vi "Get App Paths.vi"(8 "error in (no error)":errorcluster, 11 "Build Name":string) -> (0 "error out":errorcluster, 3 "Paths":T1)   [LabVIEW 2020, in "RTAF.lvlib"]
doc: "This VI returns the root directory of the main VI.\n\nIf the system is running as an executable it returns the directory the exe resides in."
uses:
  RTAF.lvlib
  App Paths.ctl
  <userlib>/_OpenG.lib/file/file.llb/Convert File Extension (Path)__ogtk.vi
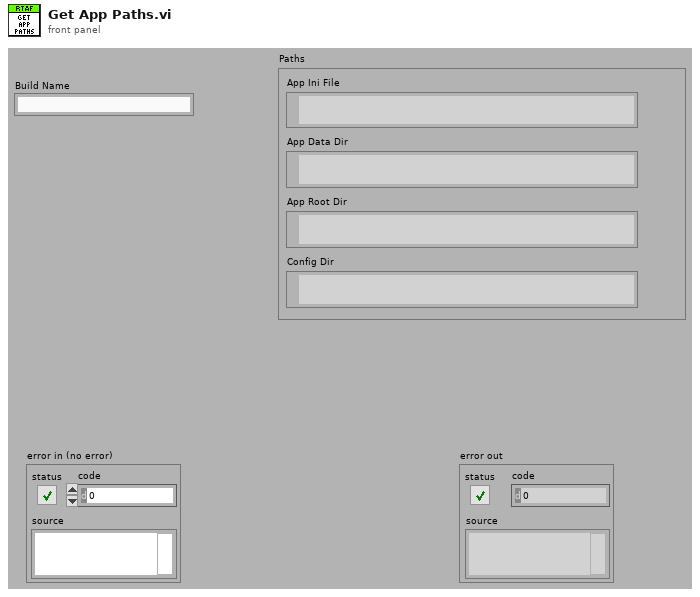
[diagram p1: front panel]
types:
  T1 = typedef "RTAF.lvlib/App Paths.ctl" = cluster{"App Ini File":path, "App Data Dir":path, "Config Dir":path, "App Root Dir":path}
  T2 = enum32{"invalid app kind", "Development System", "Run Time System", "Student Edition", "Embedded LabVIEW", "Evaluation", "Custom"}
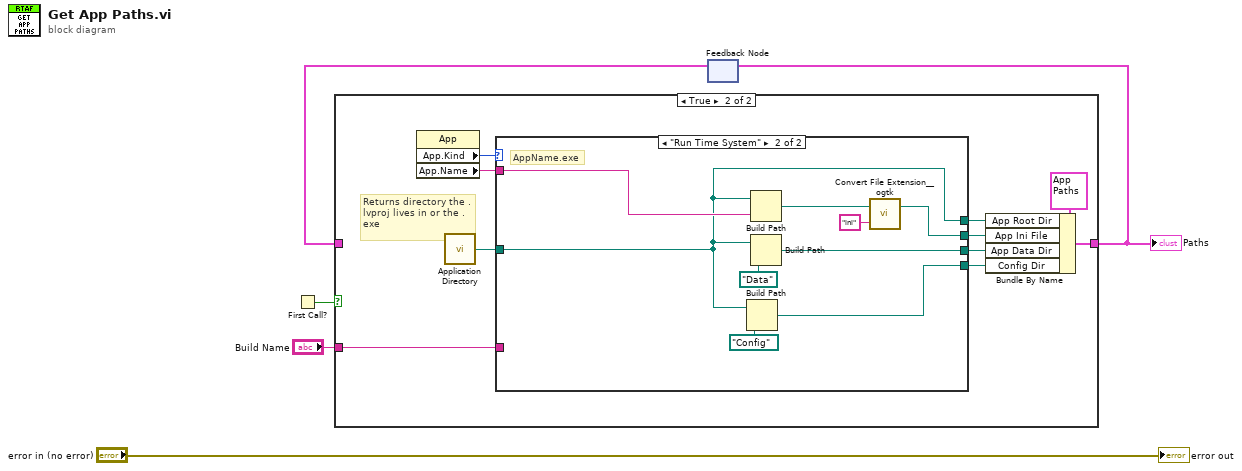
[diagram p0: block diagram]
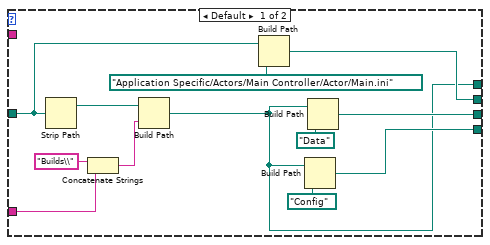
[diagram p3: hidden frame]
diagram:
  n1 = First Call?() -> (First Call?: T/F=w5:bool)
  n2 = feedback #1() -> (w3:T1)  [unwired: 1 in]
  n3 = case shown="True" w5 {
    tunnel: [w6 w16] -> w4
    tunnel: w3 -> [w6 _]
    tunnel: "Build Name" -> [_ w7]
    frame False {
    }
    frame True {
      # "Returns directory the .lvproj lives in or the .exe"
      n4 = property class="App"() -> ("App.Kind"=w12:T2, "App.Name"=w14:string)  [unwired: 2 in, 2 out]
      n5 = call <vilib>:"Application Directory.vi"() -> ("Application Directory"=w13:path)
      n6 = case shown="\"Run Time System\"" w12 {
        tunnel: [w26 w37] -> w10
        tunnel: w13 -> [w21 w29]
        tunnel: w14 -> [_ w30]
        tunnel: [w24 w34] -> w9
        tunnel: [w22 w31] -> w11
        tunnel: [w20 w29] -> w8
        tunnel: w7 -> [w17 _]
        frame Default {
          n7 = Strip Path(path=w21) -> (stripped path=w28:path)  [unwired: 1 out]
          n8 = Concatenate Strings("Builds\\" ("string"), w17) -> (w18:string)
          n9 = Build Path(base path=w28, name or relative path=w18) -> (appended path=w20:path)
          n10 = Build Path(base path=w21, name or relative path=path "Application Specific/Actors/Main Controller/Actor/Main.ini") -> (appended path=w22:path)
          n11 = Build Path(base path=w20, name or relative path=path "Config") -> (appended path=w24:path)
          n12 = Build Path(base path=w20, name or relative path=path "Data") -> (appended path=w26:path)
        }
        frame "Run Time System" {
          # "AppName.exe"
          n13 = Build Path(base path=w29, name or relative path=path "Config") -> (appended path=w34:path)
          n14 = Build Path(base path=w29, name or relative path=w30) -> (appended path=w33:path)
          n15 = Build Path(base path=w29, name or relative path=path "Data") -> (appended path=w37:path)
          n16 = call-poly <userlib>:"Convert File Extension__ogtk.vi"("new ending (none)"="ini", "file name"=w33) -> ("new filename"=w31:path)  [unwired: 1 out]
        }
      }
      n17 = Bundle By Name(cluster=T1 {"App Ini File"=path "C:/Dropbox/pgsserver/dev/Framework/source/Modules/Main", "App Data Dir"=path "C:/Dropbox/pgsserver/dev/Framework/source/Modules/Main/Main.ini", "Config Dir"=path "C:/Dropbox/pgsserver/dev/Framework/Builds/App/Data", "App Root Dir"=path ""} ("Paths"), "App Root Dir"=w8, "App Ini File"=w11, "App Data Dir"=w10, "Config Dir"=w9) -> (w16:T1)
    }
  }
  "Paths" <- w4
  n18 = feedback-in #1(w4) -> ()
  "error out" <- "error in (no error)"
